vi "GetType.vi"(8 "error in (no error)":errorcluster, 11 "Create Channel Arbitrary Waveform I16 [ACH] Msg":refnum<class "Create Channel Arbitrary Waveform I16 [ACH] Msg.lvclass">) -> (0 "error out":errorcluster, 2 "Data Sample":variant, 3 "Create Channel Arbitrary Waveform I16 [ACH] Msg":refnum<class "Create Channel Arbitrary Waveform I16 [ACH] Msg.lvclass">)   [LabVIEW 2016, in "CS++Fgen.lvlib" / "Create Channel Arbitrary Waveform I16 [ACH] Msg.lvclass"]
doc: "This VI delivers a sample of the data type format the message expects."
uses:
  Create Channel Arbitrary Waveform I16 [ACH] Msg.lvclass
  Create Channel Arbitrary Waveform I16 [ACH] Msg.lvclass/Create Channel Arbitrary Waveform I16 [ACH] Msg.ctl
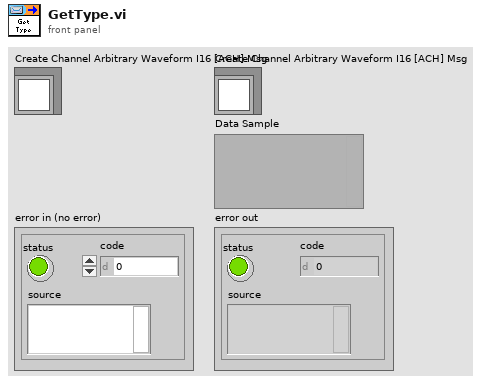
[diagram p1: front panel]
types:
  T1 = cluster{"Channel Name (\"\")":string, "Waveform Data Array":i16[]}
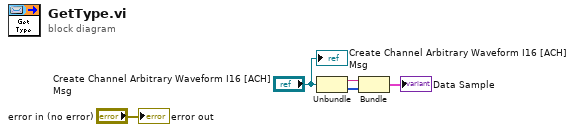
[diagram p0: block diagram]
diagram:
  n1 = Unbundle("Create Channel Arbitrary Waveform I16 [ACH] Msg") -> (w2:string, w1:i16[])
  n2 = Bundle("Channel Name (\"\")"=w2, "Waveform Data Array"=w1) -> (→"Data Sample":T1)  [unwired: 1 in]
  "error out" <- "error in (no error)"
  "Create Channel Arbitrary Waveform I16 [ACH] Msg" <- "Create Channel Arbitrary Waveform I16 [ACH] Msg"
